vi "sub_test-start-check.vi"(8 "error in":errorcluster) -> (0 "error out":errorcluster)   [LabVIEW 2019]
uses:
  _ctrl/rw.ctl
  sequence_single.ctl
  SubVIs/common/_ctrl/system-status.ctl
  _ctrl/init-r-stop.ctl
  _ctrl/create-rw-close.ctl
  Global 1.vi
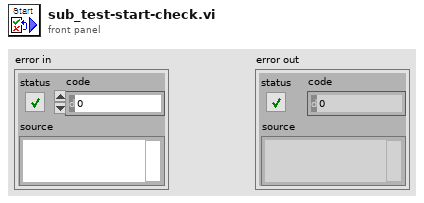
[diagram p1: front panel]
types:
  T1 = typedef "rw.ctl" = enum16{"read", "write"}
  T2 = typedef "Testing-info.ctl" = cluster{"전체채널수":u8, "현재채널번호":u8, "Irms":dbl, "입력전압":dbl, "입력전류":dbl, "출력전압":dbl, "출력전류":dbl, "온도":dbl, "제어단 단선":bool, "제어단 단락":bool, "제어단 특성변화":bool, "출력단 단선":bool, "출력단 단락":bool, "출력단 특성변화":bool, "출력단 전압":bool, "카운트 일치":bool, "Irms 판정":bool, "온도":bool, "테스트 회수":u32, "TestType":T3, "현재회수":u32, "Ch selection":cluster{"1ch":bool, "2ch":bool, "3ch":bool, "4ch":bool, "5ch":bool, "6ch":bool}, "반복":u32, "Path":path, "파일생성주기":u32, "start time":dbl, "stop time":dbl, "현재반복회수":u32, "NG":cluster{"입출력 카운트":bool, "출력전류RMS":bool}}
  T3 = typedef "sequence_single.ctl" = enum16{"Register", "RC", "B1", "B2", "B3", "Oper_LV", "Oper_HV", "ContR_LV"}
  T4 = cluster{"1ch":bool, "2ch":bool, "3ch":bool, "4ch":bool, "5ch":bool, "6ch":bool}
  T5 = typedef "init-r-stop.ctl" = enum16{"ini", "read", "stop"}
  T6 = typedef "system-status.ctl" = enum16{"Initial", "Update", "Clear", "Read"}
  T7 = typedef "create-rw-close.ctl" = enum16{"create", "write", "read", "delete", "close"}
  T8 = typedef "Test Mode.ctl" = enum32{"저항부하", "캐패시터부하", "B수명 - 1", "B수명 - 2", "B수명 - 3", "저전압모드 동작검사", "저전압모드 접촉저항", "고전압모드 동작검사"}
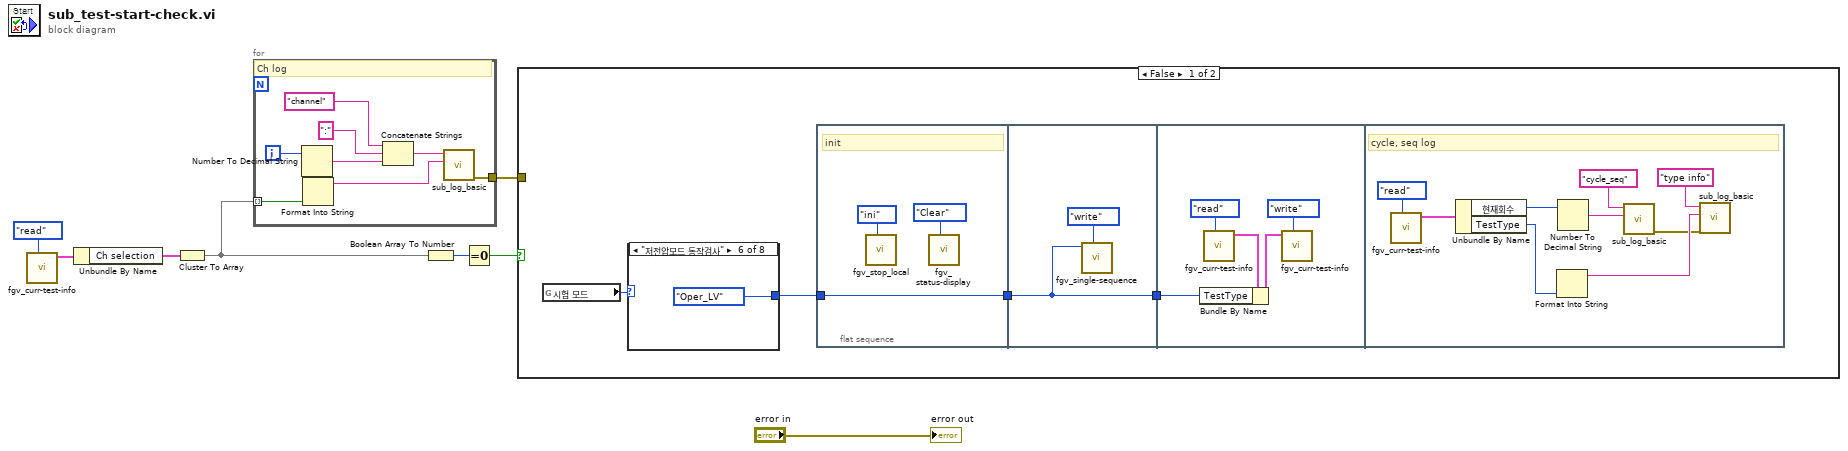
[diagram p0: block diagram]
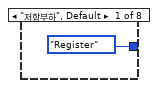
[diagram p2: hidden frame]
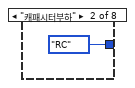
[diagram p3: hidden frame]
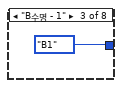
[diagram p4: hidden frame]
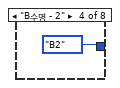
[diagram p5: hidden frame]
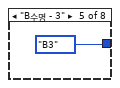
[diagram p6: hidden frame]
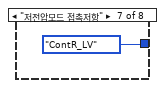
[diagram p7: hidden frame]
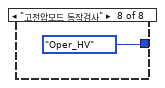
[diagram p8: hidden frame]
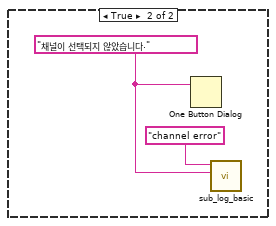
[diagram p9: hidden frame]
diagram:
  n1 = call "fgv_curr-test-info.vi"("cmd"=rw."read") -> ("현재테스트 정보 2"=w7:T2)  [unwired: 10 in]
  n2 = Unbundle By Name(w7) -> ("Ch selection"=w6:T4)
  n3 = Cluster To Array(cluster=w6) -> (array=w3:bool[])
  n4 = for {
    tunnel: w3 -> [w12] mode=indexing
    tunnel: [w9] -> w2
    i -> [w16]
    # "Ch log"
    n5 = Number To Decimal String(number=w16) -> (decimal integer string=w15:string)  [unwired: 1 in]
    n6 = Format Into String(w12) -> (resulting string=w10:string)  [unwired: 3 in, 1 out]
    n7 = Concatenate Strings("channel" ("Title"), ":" ("string"), w15) -> (w11:string)
    n8 = call "sub_log_basic.vi"("desc"=w10, "Title"=w11) -> ("error out"=w9:errorcluster)  [unwired: 9 in]
  }
  n9 = Boolean Array To Number(Boolean array=w3) -> (number=w5:u32)
  n10 = Equal To 0?(x=w5) -> (x = 0?=w4:bool)
  n11 = case shown="False" w4 {
    tunnel: w2 -> [_ _]
    frame False {
      n12 = global read "Global 1.vi" "시험 모드"() -> (w18:T8)
      n13 = case shown="\"저전압모드 동작검사\"" w18 {
        tunnel: [sequence_single."Register" ("Single sequence") sequence_single."RC" ("Single sequence") sequence_single."B1" ("Single sequence") sequence_single."B2" ("Single sequence") sequence_single."B3" ("Single sequence") sequence_single."Oper_LV" ("Single sequence") sequence_single."ContR_LV" ("Single sequence") sequence_single."Oper_HV" ("Single sequence")] -> w17
        frame "저항부하", Default {
        }
        frame "캐패시터부하" {
        }
        frame "B수명 - 1" {
        }
        frame "B수명 - 2" {
        }
        frame "B수명 - 3" {
        }
        frame "저전압모드 동작검사" {
        }
        frame "저전압모드 접촉저항" {
        }
        frame "고전압모드 동작검사" {
        }
      }
      n14 = flat-sequence {
        tunnel: w17 -> [w31]
        tunnel: [w31] -> w19
        tunnel: [w32] -> w20
        tunnel: w19 -> [w32]
        tunnel: w20 -> [w38]
        frame #0 {
          # "init"
          n15 = call "fgv_stop_local.vi"("cmd"=init-r-stop."ini") -> ()  [unwired: 9 in, 2 out]
          n16 = call "fgv_status-display.vi"("Mode"=system-status."Clear") -> ()  [unwired: 10 in, 1 out]
        }
        frame #1 {
          n17 = call "fgv_single-sequence.vi"("cmd"=create-rw-close."write", "Single sequence"=w32) -> ()  [unwired: 8 in, 2 out]
        }
        frame #2 {
          n18 = call "fgv_curr-test-info.vi"("cmd"=rw."read") -> ("현재테스트 정보 2"=w36:T2)  [unwired: 10 in]
          n19 = Bundle By Name(cluster=w36, "TestType"=w38) -> (w37:T2)
          n20 = call "fgv_curr-test-info.vi"("cmd"=rw."write", "현재테스트 정보"=w37) -> ()  [unwired: 9 in, 1 out]
        }
        frame #3 {
          # "cycle, seq log"
          n21 = call "fgv_curr-test-info.vi"("cmd"=rw."read") -> ("현재테스트 정보 2"=w44:T2)  [unwired: 10 in]
          n22 = Unbundle By Name(w44) -> ("현재회수"=w43:u32, "TestType"=w41:T3)
          n23 = Format Into String(w41) -> (resulting string=w40:string)  [unwired: 3 in, 1 out]
          n24 = Number To Decimal String(number=w43) -> (decimal integer string=w47:string)  [unwired: 1 in]
          n25 = call "sub_log_basic.vi"("desc"=w47, "Title"="cycle_seq") -> ("error out"=w39:errorcluster)  [unwired: 9 in]
          n26 = call "sub_log_basic.vi"("error in"=w39, "desc"=w40, "Title"="type info") -> ()  [unwired: 8 in, 1 out]
        }
      }
    }
    frame True {
      w48 = "채널이 선택되지 않았습니다." ("message")
      n27 = One Button Dialog(message=w48) -> ()  [unwired: 1 in, 1 out]
      n28 = call "sub_log_basic.vi"("desc"=w48, "Title"="channel error") -> ()  [unwired: 9 in, 1 out]
    }
  }
  "error out" <- "error in"
